vi "Disabled.vi"(7 "Robot Mode":T2, 10 "Match Info":T1={"Autonomous Elapsed Seconds"=0.0, "TeleOp Elapsed Seconds"=0.0, "Disabled Elapsed Seconds"=0.0, "Visited Autonomous"=FALSE, "Visited TeleOp"=FALSE, "Visited Disabled"=FALSE, "Autonomous Settings"={"Autonomous Style"=enum."Independent", "VI Refnum"=refnum}}, 11 "Call Context":T3) -> ()   [LabVIEW 2015]
doc: "This VI is called each time a disabled packet is received from the DS. It is often used to prepare for the next robot mode, to calibrate sensors, etc."
uses:
  <vilib>/Rock Robotics/WPI/DriverStation/WPI_DriverStationDerivedRobotMode.ctl
  <vilib>/Rock Robotics/WPI/DriverStation/WPI_DriverStationRobotMode2.ctl
  <vilib>/Rock Robotics/WPI/DriverStation/WPI_DriverStationMatch Info.ctl
  <vilib>/Rock Robotics/WPI/Utilities/WPI_GetSetVariantRefNum.vi
  <vilib>/Rock Robotics/Network Tables/NT Read Boolean.vi
  <vilib>/Rock Robotics/Network Tables/NT Read Number.vi
  Robot Global Data.vi
  <vilib>/Rock Robotics/Network Tables/NT Write String.vi
panel:
  out "lifter":dbl
  in  "Reset encoder":bool
  out "Valid Target Obtained":bool
  out "Pitch Degrees to Center":dbl
  out "Horizontal Degrees to Center":dbl
  out "Pitch (Degrees)":dbl
  out "Right Drive":dbl
  out "Left Drive":dbl
  out "Pitch (Encoder Counts)":dbl
  out "Value Sequence":dbl[][](array[numeric])
  out "Type Sequence":string[][](array[string])
  out "Selected Script":string
  out "Script Path":string
  out "filenames":string[](array[string])
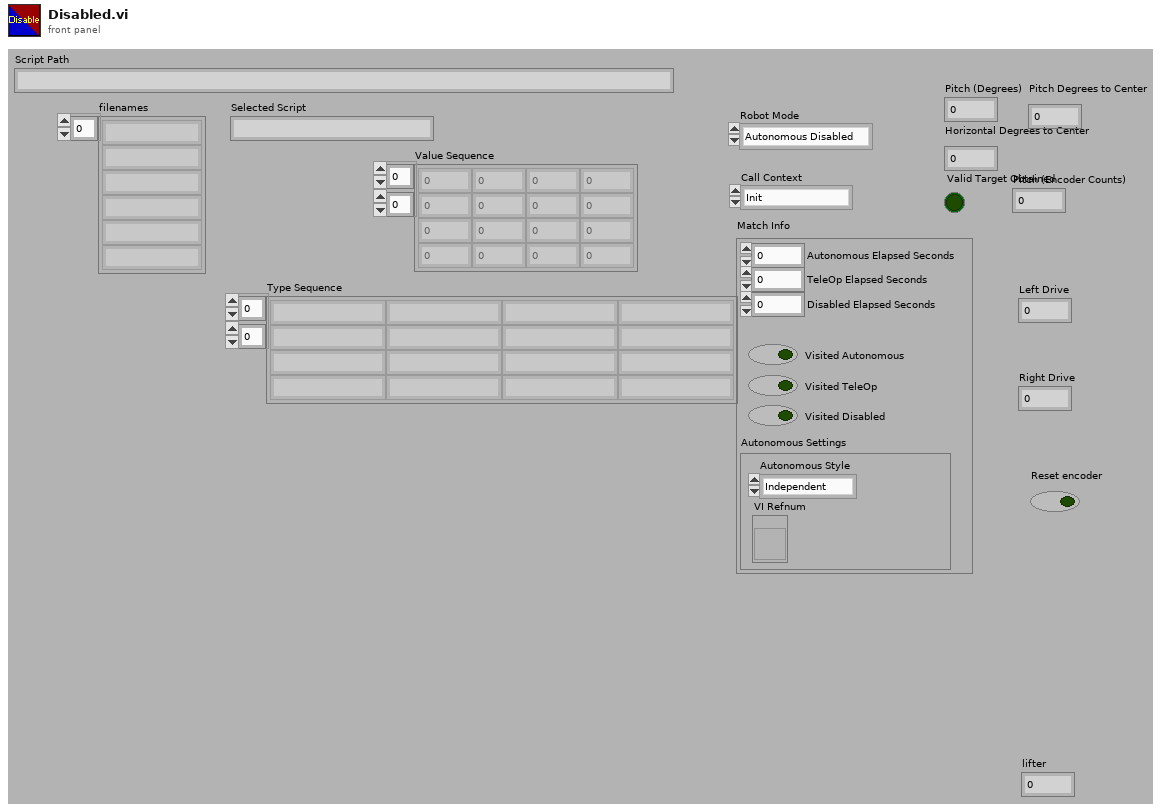
[diagram p1: front panel]
types:
  T1 = typedef "WPI_DriverStationMatch Info.ctl" = cluster{"Autonomous Elapsed Seconds":dbl, "TeleOp Elapsed Seconds":dbl, "Disabled Elapsed Seconds":dbl, "Visited Autonomous":bool, "Visited TeleOp":bool, "Visited Disabled":bool, "Autonomous Settings":cluster{"Autonomous Style":enum16{"Iterative", "Independent"}, "VI Refnum":refnum<vi>}}
  T2 = typedef "WPI_DriverStationRobotMode2.ctl" = enum16{"Autonomous Disabled", "Autonomous Enabled", "Teleop Disabled", "Teleop Enabled", "Disconnected", "Finish", "Test Disabled", "Test Enabled", "Emergency Stopped"}
  T3 = typedef "WPI_DriverStationDerivedRobotMode.ctl" = enum16{"Init", "Execute", "Stop"}
  T4 = typedef "WPI_MotorControlDeviceRef.ctl" = cluster{"DeviceStatus":errorcluster, "Type":T5, "PWM":cluster{"PWM Channel":T6, "DeadBand":T7}, "CAN":cluster{"Device Number":u8, "Control Mode":T8, "Semaphore":T9, "Max Vout":dbl, "TalonSRX Control Mode":T10}, "Invert":bool}
  T5 = typedef "WPI_MotorControlType.ctl" = enum16{"PWM", "CAN", "CANTalonSRX"}
  T6 = typedef "FPGA_DIOPWMChannel.ctl" = enum8{"PWM 0", "PWM 1", "PWM 2", "PWM 3", "PWM 4", "PWM 5", "PWM 6", "PWM 7", "PWM 8", "PWM 9", "PWM MXP 0", "PWM MXP 1", "PWM MXP 2", "PWM MXP 3", "PWM MXP 4", "PWM MXP 5", "PWM MXP 6", "PWM MXP 7", "PWM MXP 8", "PWM MXP 9", "Invalid"}
  T7 = typedef "WPI_PWMDeadband.ctl" = cluster{"Name":string, "maxPositivePwm":i32, "minPositivePwm":i32, "centerPwm":i32, "maxNegativePwm":i32, "minNegativePwm":i32, "angularRange":u16}
  T8 = typedef "WPI_CANJaguar_ControlMode.ctl" = enum8{"Percent VBus", "Current", "Speed", "Position", "Voltage"}
  T9 = typedef "Semaphore RefNum" = refnum<k1>
  T10 = typedef "WPI_CANTalonSRX_APIControlMode.ctl" = enum8{"Percent VBus", "Speed", "Position", "Slave", "Unchanged / Invalid", "Voltage Compensation", "Current", "Motion Profile"}
  T11 = typedef "WPI_JoystickDevRef.ctl" = cluster{"Device":T12}
  T12 = typedef "WPI_JoystickDeviceEnum.ctl" = enum16{"USB 0", "USB 1", "USB 2", "USB 3", "USB 4", "USB 5"}
  T13 = typedef "WPI_CANTalonSRX_GlobalStatus.ctl" = cluster{"Applied Throttle":dbl, "Module Enabled":bool, "CAN Error":errorcluster, "Closed Loop Error":dbl, "Forward Limit Switch Closed":bool, "Reverse Limit Switch Closed":bool, "Sensor Position":dbl, "Sensor Velocity":dbl, "Current":dbl, "Sticky Fault - Over Temp":bool, "Sticky Fault - Under Voltage":bool, "Sticky Fault - Forward Limit":bool, "Sticky Fault - Reverse Limit":bool, "Sticky Fault - Forward Soft Limit":bool, "Sticky Fault - Reverse Soft Limit":bool, "Brake is Enabled":bool, "Encoder Position":dbl, "Encoder Velocity":dbl, "Encoder Index Count":dbl, "Encoder A Pin State":bool, "Encoder B Pin State":bool, "Encoder Index Pin State":bool, "Analog In":dbl, "Analog In Velocity":dbl, "Temperature (C)":dbl, "Battery Voltage":dbl, "Control 5 Is Supported":bool, "Current Profile Slot Select":dbl, "Pos Div 8":bool, "Vel Div 4":bool, "Pulse Width Position":i32, "Pulse Width Velocity":i32, "Pulse Width Rise To Rise (us)":i32, "Pulse Width Rise To Fall (us)":i32, "Mot Prof Active Is Under Run":bool, "Mot Prof Active Has Under Run":bool, "Mot Prof Active Is Last":bool, "Mot Prof Active Velocity Only":bool, "Mot Prof Active Is Valid":bool, "Mot Prof Buffer Is Full":bool, "Mot Prof Active Profile Slot Select":i32, "Mot Prof NextID":i32, "Mot Prof Count":i32, "Mot Prof Active Velocity":dbl, "Mot Prof Active Position":dbl, "Mot Prof Output Enable":i32}
  T14 = cluster{"Paramter Type":string[], "Parameter Values":dbl[]}
  T15 = cluster{"Type Sequence":string[][], "Value Sequence":dbl[][]}
  T16 = cluster{"Auton Index":i32[], "Auton Name":string[]}
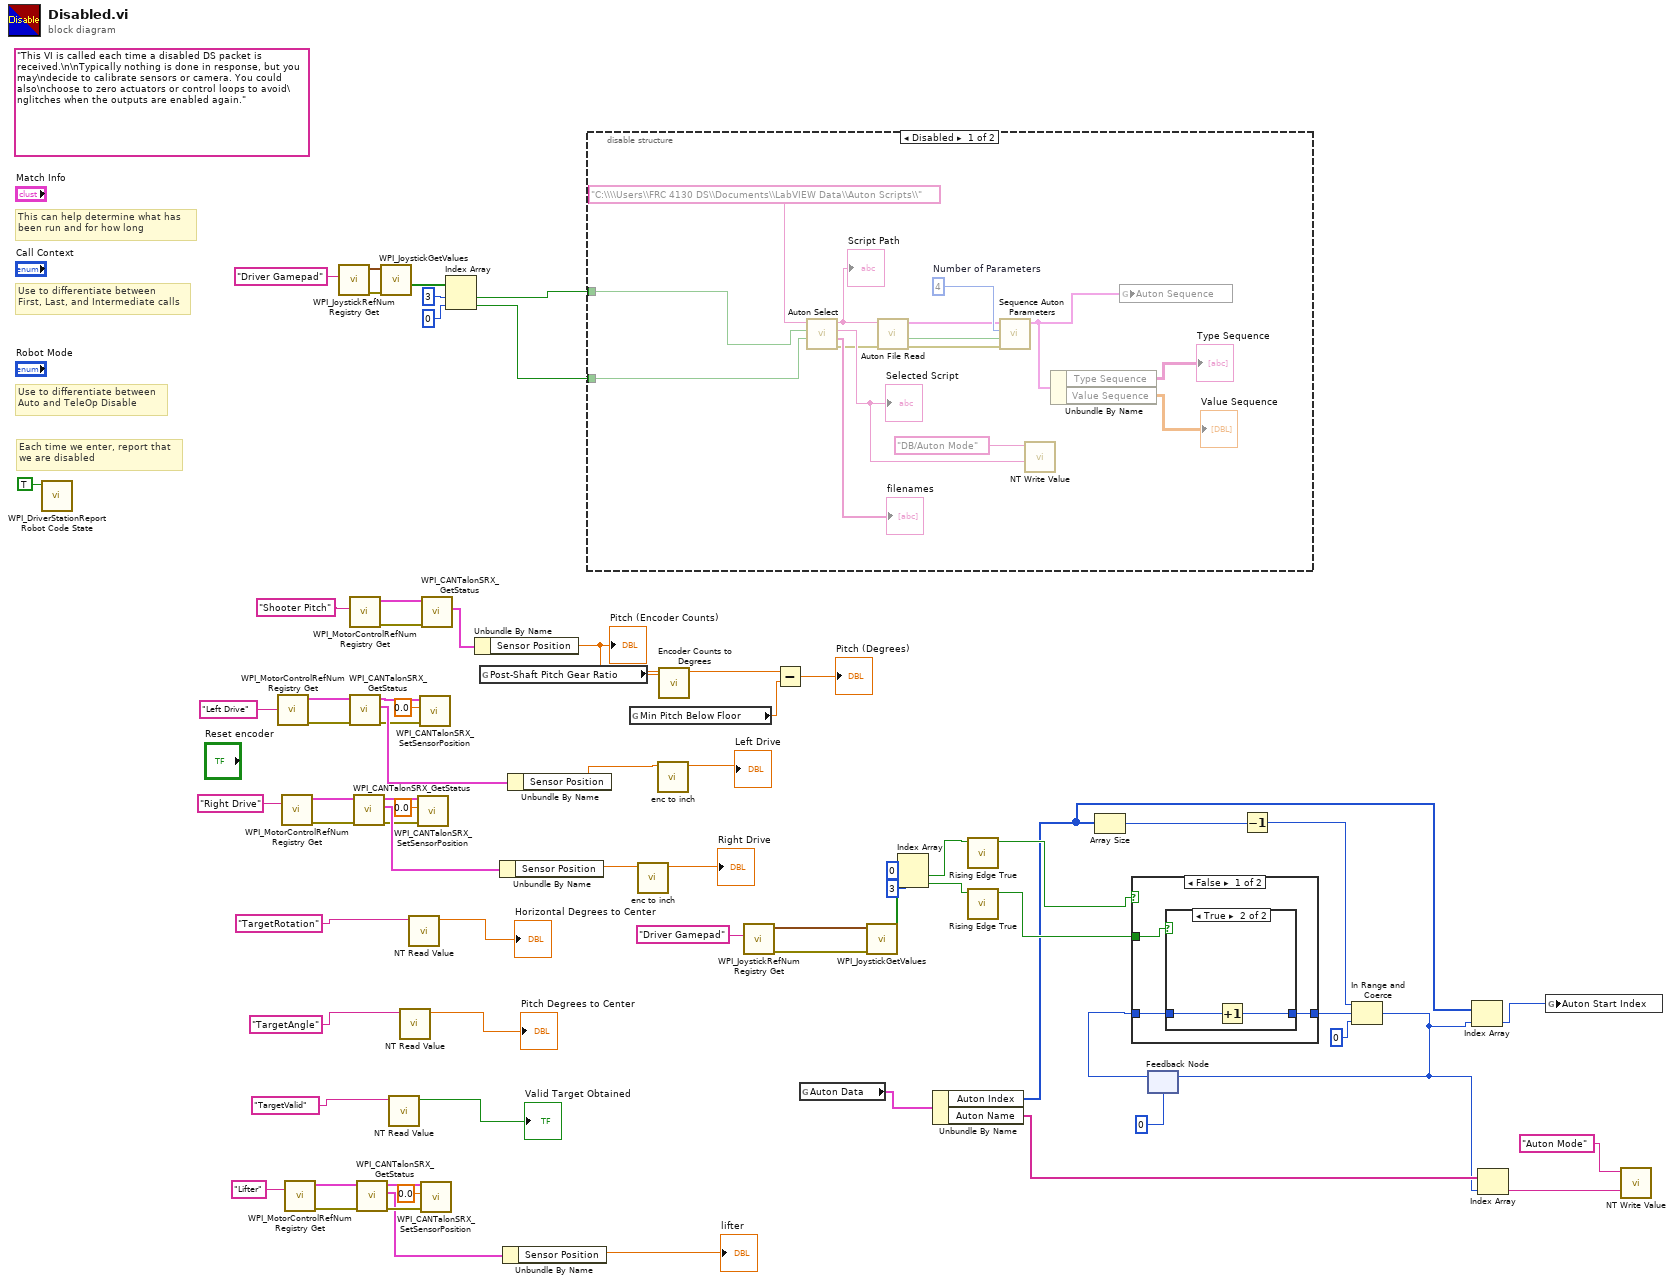
[diagram p0: block diagram]
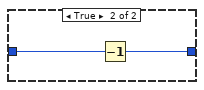
[diagram p3: hidden frame]
diagram:
  (unwired) "This VI is called each time a disabled DS packet is received.\n\nTypically nothing is done in response, but you may\ndecide to calibrate sensors or camera. You could also\nchoose to zero actuators or control loops to avoid\nglitches when the outputs are enabled again."
  # "Each time we enter, report that\nwe are disabled"
  # "Use to differentiate between\nFirst, Last, and Intermediate calls"
  # "This can help determine what has\nbeen run and for how long"
  # "Use to differentiate between\nAuto and TeleOp Disable"
  n1 = call <vilib>:"WPI_DriverStationReport Robot Code State.vi"("Disabled"=TRUE ("Autonomous")) -> ()  [unwired: 10 in, 1 out]
  n2 = call <vilib>:"WPI_MotorControlRefNum Registry Get.vi"("refnum name"="Left Drive") -> ("error out"=w59:errorcluster, "MotorControlDevRef"=w58:T4)  [unwired: 9 in]
  n3 = call <vilib>:"WPI_MotorControlRefNum Registry Get.vi"("refnum name"="Right Drive") -> ("error out"=w55:errorcluster, "MotorControlDevRef"=w56:T4)  [unwired: 9 in]
  n4 = call <vilib>:"WPI_MotorControlRefNum Registry Get.vi"("refnum name"="Lifter") -> ("error out"=w3:errorcluster, "MotorControlDevRef"=w2:T4)  [unwired: 9 in]
  n5 = call <vilib>:"WPI_JoystickRefNum Registry Get.vi"("refnum name"="Driver Gamepad") -> ("error out"=w71:errorcluster, "JoystickDevRef"=w70:T11)  [unwired: 9 in]
  n6 = call <vilib>:"WPI_MotorControlRefNum Registry Get.vi"("refnum name"="Shooter Pitch") -> ("error out"=w62:errorcluster, "MotorControlDevRef"=w63:T4)  [unwired: 9 in]
  n7 = call <vilib>:"WPI_CANTalonSRX_GetStatus.vi"("error in (no error)"=w59, "CAN Talon SRX Ref"=w58) -> ("error out"=w34:errorcluster, "Talon SRX Status"=w60:T13, "CAN Talon SRX Ref"=w35:T4)  [unwired: 7 in]
  n8 = call <vilib>:"WPI_CANTalonSRX_GetStatus.vi"("error in (no error)"=w55, "CAN Talon SRX Ref"=w56) -> ("error out"=w37:errorcluster, "Talon SRX Status"=w54:T13, "CAN Talon SRX Ref"=w36:T4)  [unwired: 7 in]
  n9 = call <vilib>:"WPI_CANTalonSRX_GetStatus.vi"("error in (no error)"=w3, "CAN Talon SRX Ref"=w2) -> ("error out"=w6:errorcluster, "Talon SRX Status"=w4:T13, "CAN Talon SRX Ref"=w7:T4)  [unwired: 7 in]
  n10 = call <vilib>:"WPI_JoystickGetValues.vi"("error in (no error)"=w71, "JoystickDevRef"=w70) -> ("Buttons"=w69:bool[])  [unwired: 5 in, 4 out]
  n11 = call-poly <vilib>:"NT Read Value.vi"("Name"="TargetValid") -> ("Boolean"=→"Valid Target Obtained":bool)  [unwired: 9 in, 1 out]
  n12 = call-poly <vilib>:"NT Read Value.vi"("Name"="TargetAngle") -> ("Numeric"=→"Pitch Degrees to Center":dbl)  [unwired: 9 in, 1 out]
  n13 = call-poly <vilib>:"NT Read Value.vi"("Name"="TargetRotation") -> ("Numeric"=→"Horizontal Degrees to Center":dbl)  [unwired: 9 in, 1 out]
  n14 = call <vilib>:"WPI_CANTalonSRX_SetSensorPosition.vi"("error in (no error)"=w37, "New Sensor Position"=0.0, "CAN Talon SRX Ref"=w36) -> ()  [unwired: 7 in, 2 out]
  n15 = call <vilib>:"WPI_CANTalonSRX_SetSensorPosition.vi"("error in (no error)"=w34, "New Sensor Position"=0.0, "CAN Talon SRX Ref"=w35) -> ()  [unwired: 7 in, 2 out]
  n16 = call <vilib>:"WPI_CANTalonSRX_SetSensorPosition.vi"("error in (no error)"=w6, "New Sensor Position"=0.0, "CAN Talon SRX Ref"=w7) -> ()  [unwired: 7 in, 2 out]
  n17 = call <vilib>:"WPI_CANTalonSRX_GetStatus.vi"("error in (no error)"=w62, "CAN Talon SRX Ref"=w63) -> ("Talon SRX Status"=w61:T13)  [unwired: 7 in, 2 out]
  n18 = Index Array(array=w69, index #1=3 ("index"), index #2=0 ("index")) -> (element #1=w66:bool, element #2=w65:bool)
  n19 = Unbundle By Name(w61) -> ("Sensor Position"=w52:dbl)
  "Pitch (Encoder Counts)" <- w52
  n20 = global read "Robot Global Data.vi" "Post-Shaft Pitch Gear Ratio"() -> (w51:dbl)
  n21 = Unbundle By Name(w54) -> ("Sensor Position"=w39:dbl)
  n22 = Unbundle By Name(w4) -> ("Sensor Position"=→"lifter":dbl)
  n23 = Unbundle By Name(w60) -> ("Sensor Position"=w41:dbl)
  n24 = disable-structure shown="Disabled" {
    disable-tunnel: w66 -> [w81 _]
    disable-tunnel: w65 -> [w80 _]
    frame Disabled {
      w85 = 4  # Number of Parameters
      n25 = call "Auton Select.vi"("Select Previous"=w80, "Select Next"=w81, "Script Folder Path"="C:\\\\Users\\FRC 4130 DS\\Documents\\LabVIEW Data\\Auton Scripts\\" ("string")) -> ("error out"=w75:errorcluster, "filenames"=→"filenames":string[], "Selected Script"=w78:string, "Script Path"=w86:string)  [unwired: 5 in]
      "Script Path" <- w86
      "Selected Script" <- w78
      n26 = call "Auton File Read.vi"("error in (no error)"=w75, "Script Path"=w86) -> ("error out"=w74:errorcluster, "New Script Loaded"=w76:bool, "Auton Parameters"=w84:T14)  [unwired: 7 in]
      n27 = call "Sequence Auton Parameters.vi"("error in (no error)"=w74, "Parse Parameters?"=w76, "Number of Parameters"=w85, "Auton Parameters"=w84) -> ("Auton Sequence"=w79:T15)  [unwired: 6 in, 1 out]
      n28 = call-poly <vilib>:"NT Write Value.vi"("String"=w78, "Name"="DB/Auton Mode") -> ()  [unwired: 9 in, 1 out]
      n29 = Unbundle By Name(w79) -> ("Type Sequence"=→"Type Sequence":string[][], "Value Sequence"=→"Value Sequence":dbl[][])
      n30 = global write "Robot Global Data.vi" "Auton Sequence"(w79) -> ()
    }
    frame Enabled {
    }
  }
  n31 = global read "Robot Global Data.vi" "Min Pitch Below Floor"() -> (w48:dbl)
  n32 = call "enc to inch.vi"("Sensor position"=w39) -> ("Inches"=→"Right Drive":dbl)  [unwired: 10 in]
  n33 = call "enc to inch.vi"("Sensor position"=w41) -> ("Inches"=→"Left Drive":dbl)  [unwired: 10 in]
  n34 = call "Encoder Counts to Degrees.vi"("Post-Shaft Gear Ratio"=w51, "Encoder Rotations"=w52) -> ("Degrees"=w50:dbl)  [unwired: 9 in]
  n35 = call <vilib>:"WPI_JoystickRefNum Registry Get.vi"("refnum name"="Driver Gamepad") -> ("error out"=w19:errorcluster, "JoystickDevRef"=w21:T11)  [unwired: 1 in, 8 out]
  n36 = Subtract(x=w50, y=w48) -> (x-y=→"Pitch (Degrees)":dbl)
  n37 = global read "Robot Global Data.vi" "Auton Data"() -> (w31:T16)
  n38 = call <vilib>:"WPI_JoystickGetValues.vi"("error in (no error)"=w19, "JoystickDevRef"=w21) -> ("Buttons"=w18:bool[])  [unwired: 5 in, 4 out]
  n39 = Index Array(array=w18, index #1=0 ("index"), index #2=3 ("index")) -> (element #1=w15:bool, element #2=w13:bool)
  n40 = Unbundle By Name(w31) -> ("Auton Index"=w11:i32[], "Auton Name"=w24:string[])
  n41 = call "Rising Edge True.vi"("Input"=w15) -> ("Output"=w14:bool)  [unwired: 10 in]
  n42 = call "Rising Edge True.vi"("Input"=w13) -> ("Output"=w12:bool)  [unwired: 10 in]
  n43 = Array Size(array=w11) -> (size(s)=w27:i32)
  n44 = feedback #1(0) -> (w29:i32)
  n45 = case shown="False" w14 {
    tunnel: w29 -> [w91 w96]
    tunnel: [w90 w95] -> w28
    tunnel: w12 -> [w89 _]
    frame False {
      n46 = case shown="True" w89 {
        tunnel: w91 -> [w92 w94]
        tunnel: [w92 w93] -> w90
        frame False {
        }
        frame True {
          n47 = Increment(x=w94) -> (x+1=w93:i32)
        }
      }
    }
    frame True {
      n48 = Decrement(x=w96) -> (x-1=w95:i32)
    }
  }
  n49 = Decrement(x=w27) -> (x-1=w26:i32)
  n50 = In Range and Coerce(upper limit=w26, x=w28, lower limit=0) -> (coerced(x)=w10:i32)  [unwired: 1 out]
  n51 = feedback-in #1(w10) -> ()
  n52 = Index Array(array=w11, index=w10) -> (element=w9:i32)
  n53 = Index Array(array=w24, index=w10) -> (element=w23:string)
  n54 = global write "Robot Global Data.vi" "Auton Start Index"(w9) -> ()
  n55 = call-poly <vilib>:"NT Write Value.vi"("String"=w23, "Name"="Auton Mode") -> ()  [unwired: 9 in, 1 out]
